vi "Shooter Teleop.vi"(10 "D-Pad":i16[](array[numeric]), 11 "Buttons":bool[](array[boolean])) -> ()   [LabVIEW 2019]
uses:
  c42b3440-6ec2-456f-9881-3dbc4d15ed6d.vi
panel:
  out "Sensor Position":dbl
  in  "270":cluster{dbl, dbl, dbl}={-8.0, 0.0, 2750.0}
  in  "180":cluster{dbl, dbl, dbl}={0.0, 0.0, 3250.0}
  in  "90":cluster{dbl, dbl, dbl}={-14.0, 0.0, 3500.0}
  in  "0":cluster{dbl, dbl, dbl}={-0.5, 0.0, 0.0}
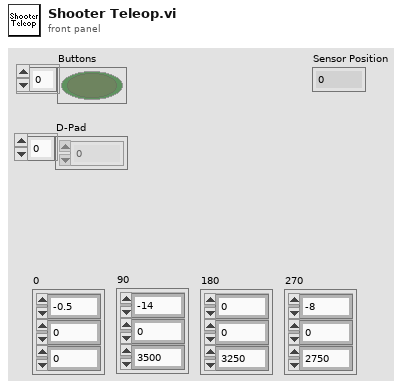
[diagram p1: front panel]
types:
  T1 = typedef "WPI_MotorControlDeviceRef.ctl" = cluster{"DeviceStatus":errorcluster, "Type":T2, "PWM":cluster{"PWM Channel":T3, "DeadBand":T4}, "CAN":cluster{"Device Number":u8, "SetOutput VI Ref":variant, "GetOutput VI Ref":variant, "Enable VI Ref":variant, "Disable VI Ref":variant, "Data":variant}, "Invert":bool, "DIO PWM":cluster{"PWM \"Enable\" Channel":T3, "DIOChannel":T5, "PWM Rate":dbl}}
  T2 = typedef "WPI_MotorControlType.ctl" = enum16{"PWM", "CAN", "DIO PWM"}
  T3 = typedef "FPGA_DIOPWMChannel.ctl" = enum8{"PWM 0", "PWM 1", "PWM 2", "PWM 3", "PWM 4", "PWM 5", "PWM 6", "PWM 7", "PWM 8", "PWM 9", "PWM MXP 0", "PWM MXP 1", "PWM MXP 2", "PWM MXP 3", "PWM MXP 4", "PWM MXP 5", "PWM MXP 6", "PWM MXP 7", "PWM MXP 8", "PWM MXP 9", "Invalid"}
  T4 = typedef "WPI_PWMDeadband.ctl" = cluster{"Name":string, "maxPositivePwm":i32, "minPositivePwm":i32, "centerPwm":i32, "maxNegativePwm":i32, "minNegativePwm":i32, "angularRange":u16}
  T5 = typedef "FPGA_DIOChannel.ctl" = enum8{"DIO 0", "DIO 1", "DIO 2", "DIO 3", "DIO 4", "DIO 5", "DIO 6", "DIO 7", "DIO 8", "DIO 9", "DIO MXP 0", "DIO MXP 1", "DIO MXP 2", "DIO MXP 3", "DIO MXP 4", "DIO MXP 5", "DIO MXP 6", "DIO MXP 7", "DIO MXP 8", "DIO MXP 9", "DIO MXP 10", "DIO MXP 11", "DIO MXP 12", "DIO MXP 13", "DIO MXP 14", "DIO MXP 15", "SPI Port CS1", "SPI Port CS2", "SPI Port CS3", "SPI Port MISO", "SPI Port MOSI", "Invalid"}
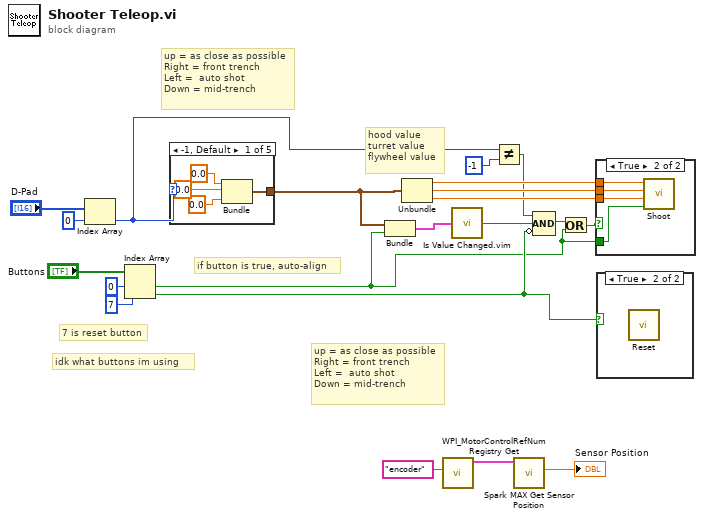
[diagram p0: block diagram]
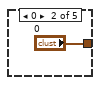
[diagram p4: hidden frame]
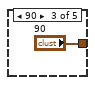
[diagram p5: hidden frame]
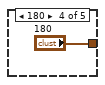
[diagram p6: hidden frame]
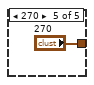
[diagram p7: hidden frame]
diagram:
  # "up = as close as possible\nRight = front trench\nLeft =  auto shot\nDown = mid-trench"
  # "up = as close as possible\nRight = front trench\nLeft =  auto shot\nDown = mid-trench"
  # "7 is reset button"
  # "if button is true, auto-align"
  # "hood value\nturret value\nflywheel value"
  # "idk what buttons im using"
  n1 = Index Array(array="D-Pad", index=0) -> (element=w6:i16)
  n2 = Index Array(array="Buttons", index #1=0 ("index"), index #2=7 ("index")) -> (element #1=w1:bool, element #2=w10:bool)
  n3 = case shown="-1, Default" w6 {
    tunnel: [w22 "0" "90" "180" "270"] -> w3
    frame -1, Default {
      n4 = Bundle(0.0, 0.0, 0.0) -> (w22:cluster{dbl, dbl, dbl})  [unwired: 1 in]
    }
    frame 0 {
    }
    frame 90 {
    }
    frame 180 {
    }
    frame 270 {
    }
  }
  n5 = Bundle("270"=w3, w1) -> (w2:cluster{"270":cluster{dbl, dbl, dbl}, bool})  [unwired: 1 in]
  n6 = Unbundle(w3) -> (w17:dbl, w16:dbl, w15:dbl)
  n7 = call <vilib>:"WPI_MotorControlRefNum Registry Get.vi"("refnum name"="encoder") -> ("MotorControlDevRef"=w8:T1)  [unwired: 9 in, 1 out]
  n8 = call "Is Value Changed.vim"("value"=w2) -> ("changed or first call?"=w13:bool)
  n9 = Not Equal?(x=w6, y=i16 -1) -> (x != y?=w12:bool)
  n10 = call <vilib>:"Spark MAX Get Sensor Position.vi"("MotorControlDevRef in"=w8) -> ("Sensor Position"=→"Sensor Position":dbl)  [unwired: 7 in, 3 out]
  n11 = Compound Arithmetic op=AND(w12, w13, invert w10) -> (w5:bool)
  n12 = Or(x=w5, y=w1) -> (x .or. y?=w4:bool)
  n13 = case shown="True" w4 {
    tunnel: w17 -> [_ w33]
    tunnel: w16 -> [_ w32]
    tunnel: w15 -> [_ w31]
    tunnel: w1 -> [_ w30]
    frame False {
      # "nothing"
    }
    frame True {
      n14 = call "Shoot.vi"("otto aline"=w30, "wheel"=w31, "turr(et)"=w32, "hood"=w33) -> ()  [unwired: 7 in, 1 out]
    }
  }
  n15 = case shown="True" w10 {
    frame False {
    }
    frame True {
      n16 = call "Reset.vi"() -> ()  [unwired: 11 in, 1 out]
    }
  }
